vi "CameraEventCache.vi"(8 "Operation":enum16{"Create", "GetRef", "Fire"}(ring), 11 "CameraEvent":T1) -> (3 "EventRef":refnum<event-registration>)   [LabVIEW 2014]
uses:
  TypeDefs/CameraEvent.ctl
  TypeDefs/Camera.ctl
  <vilib>/Utility/miscctls.llb/LV3DPointTypeDef.ctl
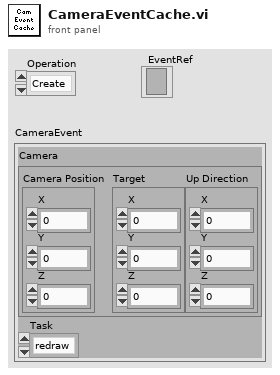
[diagram p1: front panel]
types:
  T1 = typedef "CameraEvent.ctl" = cluster{"Camera":T2, "Task":enum16{"redraw", "setTo", "setToUpdate"}}
  T2 = typedef "Camera.ctl" = cluster{"Camera Position":T3, "Target":T3, "Up Direction":T3}
  T3 = typedef "LV3DPointTypeDef.ctl" = cluster{"X":sgl, "Y":sgl, "Z":sgl}
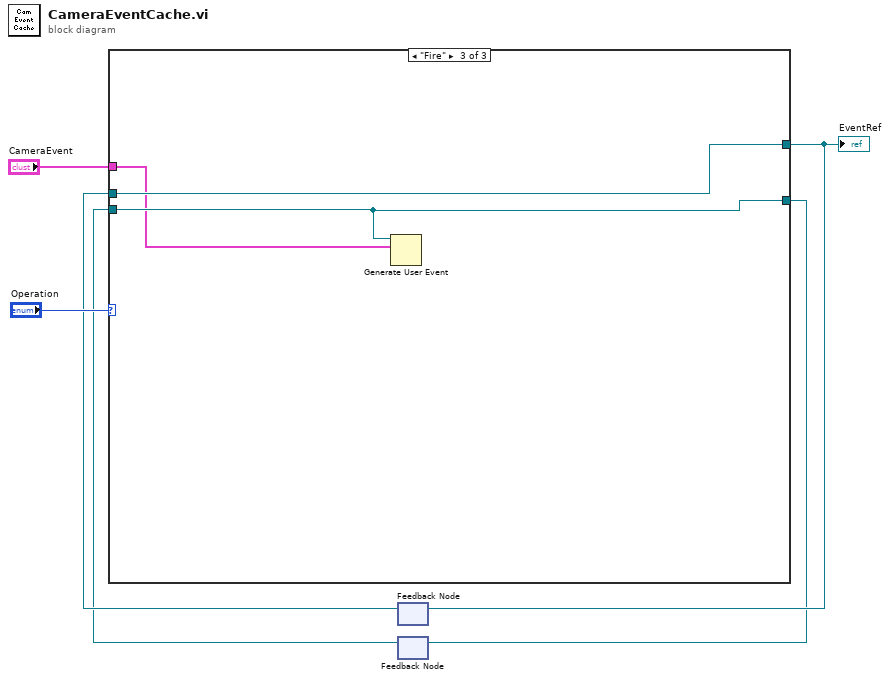
[diagram p0: block diagram]
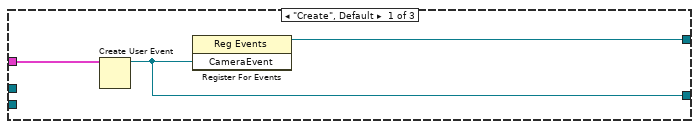
[diagram p2: hidden frame]
diagram:
  n1 = feedback #1() -> (w3:refnum<event-registration>)  [unwired: 1 in]
  n2 = feedback #2() -> (w1:refnum<user-event>)  [unwired: 1 in]
  n3 = case shown="\"Fire\"" "Operation" {
    tunnel: "CameraEvent" -> [w9 _ w12]
    tunnel: [w8 w11 w14] -> w4
    tunnel: w3 -> [_ w11 w14]
    tunnel: [w7 w10 w13] -> w2
    tunnel: w1 -> [_ w10 w13]
    frame "Create", Default {
      n4 = Create User Event(user event datatype=w9) -> (user event=w7:refnum<user-event>)  [unwired: 1 in, 1 out]
      n5 = register-events(w7) -> (reference out=w8:refnum<event-registration>)  [unwired: 2 in, 1 out]
    }
    frame "GetRef" {
    }
    frame "Fire" {
      n6 = Generate User Event(user event=w13, event data cluster=w12) -> ()  [unwired: 2 in, 2 out]
    }
  }
  "EventRef" <- w4
  n7 = feedback-in #1(w4) -> ()
  n8 = feedback-in #2(w2) -> ()
